vi "Remove Channel by Index.vi"(8 "error in (no error)":errorcluster, 10 "Channel Index":i32, 11 "CIFChannelMng in":refnum<class "CIFChannelMng.lvclass">) -> (0 "error out":errorcluster, 3 "CIFChannelMng out":refnum<class "CIFChannelMng.lvclass">)   [LabVIEW 2021, in "CIFChannelMng.lvclass"]
uses:
  CIFChannelMng.lvclass
  CIFCore/Common/CIFCoreCommon.lvlib
  CIFCore/Common/Typedef/Errors.ctl
  CIFChannels/CIFChannels.lvclass
  CIFChannels/Typedef/Channel State.ctl
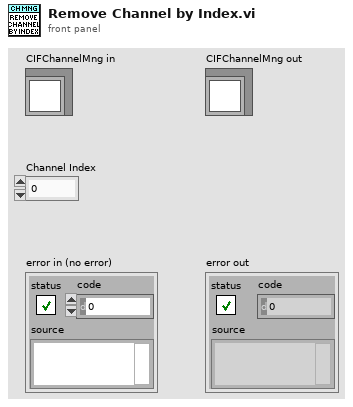
[diagram p1: front panel]
types:
  T1 = typedef "CIFCoreCommon.lvlib/Errors.ctl" = enum16{"Invalid Clock ID", "Long Sleep", "gRPC Server Not Found", "Config Parse", "Timestamp Wrap", "Delayed Execution", "Duplicate Channel", "Missing Channel", "Incorrect Type", "Flatten Error", "Unflatten Data", "Unique Name", "Plugin Not Found"}
  T2 = typedef "CIFChannels.lvclass/Channel State.ctl" = enum16{"Creating", "Disconnected", "Connecting", "Connected", "Destroyed"}
  T3 = typedef "CIFChannelMng.lvclass/Channel List for OOB.ctl" = cluster{"Name":string, "Direction":T4, "Type":string, "Connected?":bool, "Connected Name":string, "Custom Config Data":u8[], "Forced?":bool}
  T4 = typedef "CIFChannels.lvclass/Direction.ctl" = enum16{"Publisher", "Subscriber"}
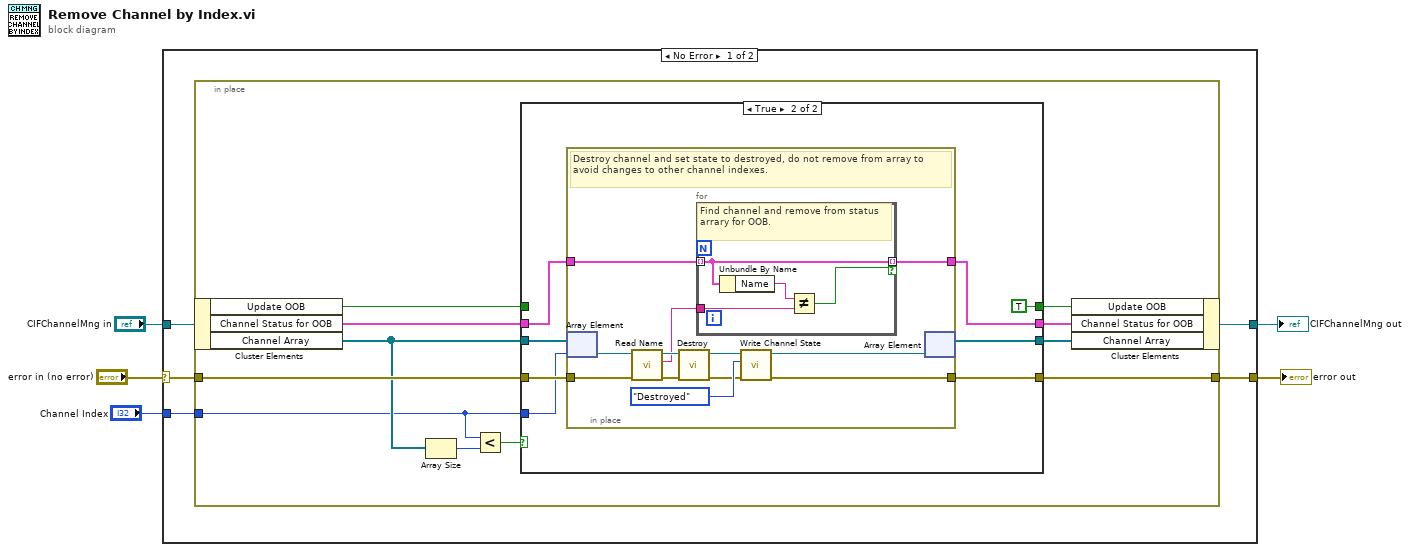
[diagram p0: block diagram]
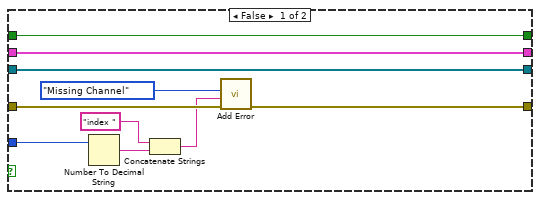
[diagram p2: hidden frame]
diagram:
  n1 = case shown="No Error" "error in (no error)" {
    selector: "error in (no error)" -> [w8 w57]
    tunnel: [w7 w57] -> w5
    tunnel: [w9 w56] -> w4
    tunnel: "CIFChannelMng in" -> [w10 w56]
    tunnel: "Channel Index" -> [w6 _]
    frame No Error {
      n2 = in-place {
        in-place-border: w8 -> [w19]
        in-place-border: [w13] -> w7
        in-place-border: w6 -> [w14]
        n3 = in-place-cluster #1(w10) -> ("Update OOB"=w12:bool, "Channel Status for OOB"=w21:T3[], "Channel Array"=w17:refnum<class "CIFChannels.lvclass">[])
        n4 = Array Size(array=w17) -> (size(s)=w16:i32)
        n5 = Less?(x=w14, y=w16) -> (x < y?=w15:bool)
        n6 = case shown="True" w15 {
          tunnel: w21 -> [w24 w34]
          tunnel: [w24 w33] -> w20
          tunnel: w19 -> [w31 w39]
          tunnel: [w25 w35] -> w18
          tunnel: [w23 w38] -> w13
          tunnel: w17 -> [w25 w37]
          tunnel: w14 -> [w29 w36]
          tunnel: w12 -> [w22 _]
          tunnel: [w22 TRUE ("Update OOB")] -> w11
          frame False {
            n7 = Number To Decimal String(number=w29) -> (decimal integer string=w27:string)  [unwired: 1 in]
            n8 = Concatenate Strings("index " ("string"), w27) -> (w26:string)
            n9 = call "Add Error.vi"("error in (no error)"=w31, "String to Append"=w26, "Error"=Errors."Missing Channel") -> ("error out"=w23:errorcluster)  [unwired: 8 in]
          }
          frame True {
            n10 = in-place {
              in-place-border: w39 -> [w51]
              in-place-border: [w50] -> w38
              in-place-border: w34 -> [w42]
              in-place-border: [w40] -> w33
              # "Destroy channel and set state to destroyed, do not remove from array to avoid changes to other channel indexes."
              n11 = in-place-array #2(w37, w36) -> (w49:refnum<class "CIFChannels.lvclass">)
              n12 = call "Read Name.vi"("error in (no error)"=w51, "CIFChannels in"=w49) -> ("error out"=w46:errorcluster, "Name"=w41:string, "CIFChannels out"=w47:refnum<class "CIFChannels.lvclass">)  [unwired: 7 in]
              n13 = call-dynamic "Destroy.vi"("error in (no error)"=w46, "CIFChannels in"=w47) -> ("error out"=w43:errorcluster, "CIFChannels out"=w44:refnum<class "CIFChannels.lvclass">)  [unwired: 8 in]
              n14 = for {
                tunnel: w42 -> [w53] mode=indexing
                tunnel: w41 -> [w54]
                tunnel: [w53] -> w40 mode=indexing if=w52
                # "Find channel and remove from status arrary for OOB."
                n15 = Unbundle By Name(w53) -> ("Name"=w55:string)
                n16 = Not Equal?(x=w55, y=w54) -> (x != y?=w52:bool)
              }
              n17 = call "Write Channel State.vi"("error in (no error)"=w43, "Channel State"=Channel_State."Destroyed", "CIFChannels in"=w44) -> ("error out"=w50:errorcluster, "CIFChannels out"=w48:refnum<class "CIFChannels.lvclass">)  [unwired: 7 in]
              n18 = in-place-array #2(w48) -> (w35:refnum<class "CIFChannels.lvclass">[])  [unwired: 1 out]
            }
          }
        }
        n19 = in-place-cluster #1("Update OOB"=w11, "Channel Status for OOB"=w20, "Channel Array"=w18) -> (w9:refnum<class "CIFChannelMng.lvclass">)
      }
    }
    frame Error {
    }
  }
  "error out" <- w5
  "CIFChannelMng out" <- w4
